vi "PicoScope4000aOpen.vi"(0 "error in (no error)":errorcluster, 1 "Serial Number":string, 2 "setProbeInteractionCallback":bool, 5 "Use Serial Number":bool, 7 "Resolution":u32(ring) items=["8-bit", "12-bit", "14-bit"], 9 "USB powered control":bool, 11 "USB 3.0 on non-USB 3.0 port control":bool) -> (4 "error out":errorcluster, 6 "handle":i16, 10 "Unit Info":T1, 12 "Max ADC value":i16, 13 "USB powered":bool, 14 "USB 3.0 on non-USB 3.0 port":bool)   [LabVIEW 2009]
doc: "This VI opens a PicoScope 3000a/b and returns a handle to the device."
uses:
  ps4000A.dll
  ps4000aWrap.dll
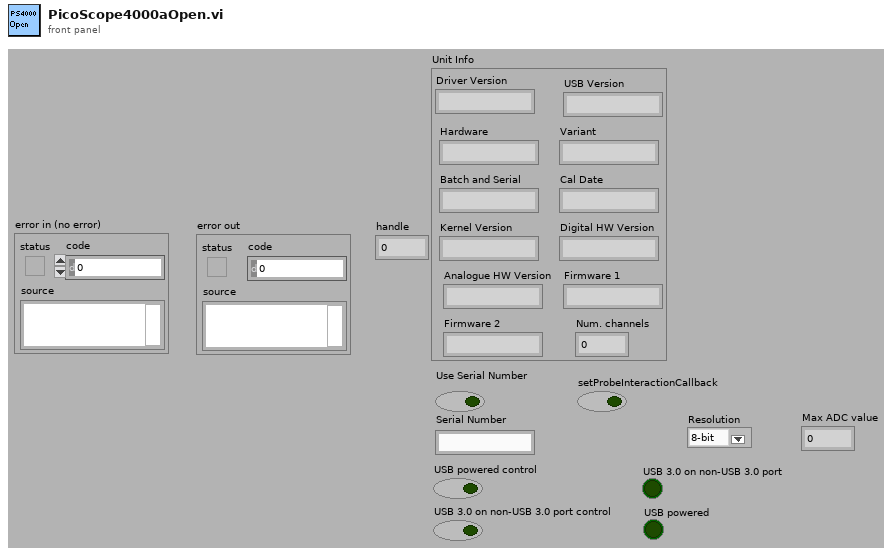
[diagram p1: front panel]
types:
  T1 = cluster{"Driver Version":string, "USB Version":string, "Hardware":string, "Variant":string, "Batch and Serial":string, "Cal Date":string, "Kernel Version":string, "Digital HW Version":string, "Analogue HW Version":string, "Firmware 1":string, "Firmware 2":string, "Num. channels":i16}
  T2 = cluster{"Driver Version":string, "USB Version":string, "Hardware":string, "Variant":string, "Batch and Serial":string, "Cal Date":string, "Kernel Version":string, "Digital HW Version":string, "Analogue HW Version":string, "Firmware 1":string, "Firmware 2":string}
  T3 = cluster{"Driver Version":string, "USB Version":string, "Hardware":string, "Variant":string, "Batch and Serial":string, "Cal Date":string, "Kernel Version":string, "Digital HW Version":string, "Analogue HW Version":string, "Firmware 1":string, "Firmware 2":string, i16}
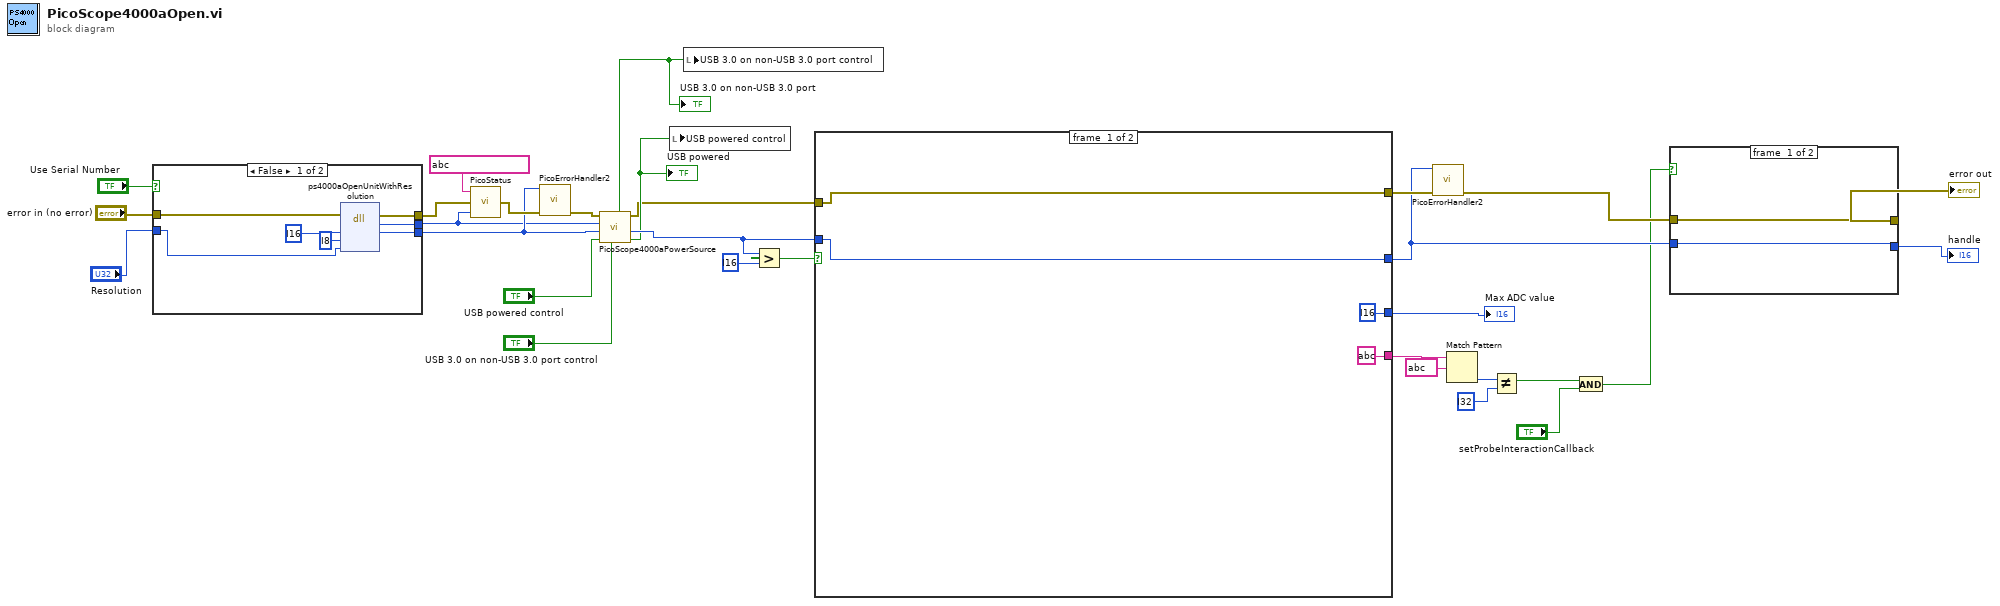
[diagram p0: block diagram]
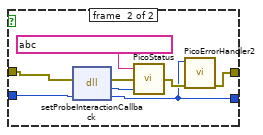
[diagram p2: hidden frame]
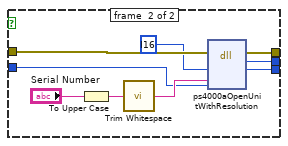
[diagram p3: hidden frame]
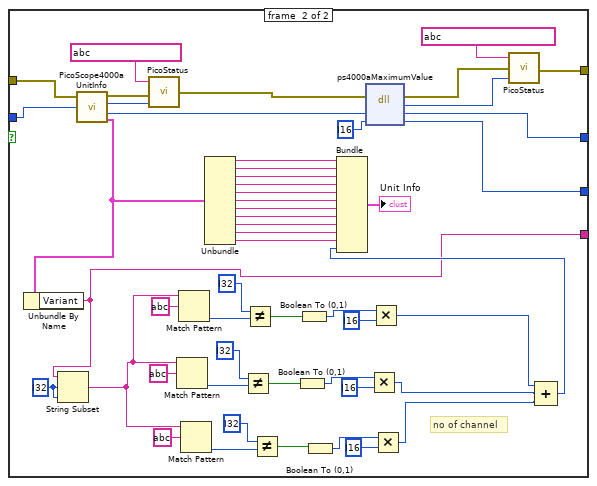
[diagram p4: hidden frame]
diagram:
  n1 = case shown="False" "Use Serial Number" {
    tunnel: "error in (no error)" -> [w37 w43]
    tunnel: [w36 w46] -> w17
    tunnel: [w35 w45] -> w15
    tunnel: [w34 w44] -> w16
    tunnel: "Resolution" -> [w31 w39]
    frame #0 {
      n2 = dll-call lib="ps4000A.dll" fn="ps4000aOpenUnitWithResolution" ("ps3000.dll:_ps3000_open_unit@0")(error in=w37, "handle"=i16 ?, "serial"=i8 ?, "resolution"=w31) -> (error out=w36:errorcluster, "PICO_STATUS"=w35:u32, "handle"=w34:i16)  [unwired: 4 in, 1 out]
    }
    frame #1 {
      n3 = To Upper Case(1:"Serial Number") -> (0:w41:string)
      n4 = call <vilib>:"Trim Whitespace.vi"("string"=w41) -> ("trimmed string"=w40:string)  [unwired: 1 in]
      n5 = dll-call lib="ps4000A.dll" fn="ps4000aOpenUnitWithResolution" ("ps3000.dll:_ps3000_open_unit@0")(error in=w43, "handle"=i16 ?, "serial"=w40, "resolution"=w39) -> (error out=w46:errorcluster, "PICO_STATUS"=w45:u32, "handle"=w44:i16)  [unwired: 4 in, 1 out]
    }
  }
  n6 = call "PicoStatus.vi"("PICO STATUS"=w15, "error in"=w17, "source"=string ?) -> ("error out"=w18:errorcluster)
  n7 = call "PicoErrorHandler2.vi"("error in (no error)"=w18, "handle In"=w16) -> ("error out"=w19:errorcluster)  [unwired: 9 in]
  n8 = call "PicoScope4000aPowerSource.vi"("USB 3.0 on non-USB 3.0 port control"="USB 3.0 on non-USB 3.0 port control", "USB powered control"="USB powered control", "handle in"=w16, "PICO STATUS IN"=w15, "error in (no error)"=w19) -> ("USB powered"=w21:bool, "handle out"=w26:i16, "error out"=w13:errorcluster, "USB 3.0 on non-USB 3.0 port"=w20:bool)  [unwired: 2 in, 1 out]
  "USB 3.0 on non-USB 3.0 port" <- w20
  "USB powered" <- w21
  n9 = local write "USB powered control"(w21) -> ()
  n10 = local write "USB 3.0 on non-USB 3.0 port control"(w20) -> ()
  n11 = Greater?(x=w26, y=i16 ?) -> (0:w29:bool)
  n12 = case shown="True" w29 {
    tunnel: w26 -> [w50 w101]
    tunnel: [w50 w57] -> w10
    tunnel: [w49 w61] -> w14
    tunnel: w13 -> [w49 w55]
    tunnel: [i16 ? ("value") w54] -> w12
    tunnel: [string ? ("Variant") w51] -> w7
    frame #0 {
    }
    frame #1 {
      w99 = i32 ? ("offset (0)")
      # "no of channel"
      n13 = call "PicoScope4000aUnitInfo.vi"("error in (no error)"=w55, "handle in"=w101) -> ("error out"=w100:errorcluster, "PICO_STATUS"=w52:u32, "handle out"=w56:i16, "Unit Info"=w98:T2)  [unwired: 1 in]
      n14 = Unbundle By Name(w98) -> ("Variant"=w51:string)
      n15 = String Subset(string=w51, offset (0)=w99, length (rest)=w99) -> (substring=w67:string)
      n16 = call "PicoStatus.vi"("PICO STATUS"=w52, "error in"=w100, "source"=string ?) -> ("error out"=w60:errorcluster)
      n17 = Match Pattern(string=w67, regular expression=string ?) -> (offset past match=w84:i32)  [unwired: 1 in, 3 out]
      n18 = Match Pattern(string=w67, regular expression=string ?) -> (offset past match=w72:i32)  [unwired: 1 in, 3 out]
      n19 = Match Pattern(string=w67, regular expression=string ?) -> (offset past match=w82:i32)  [unwired: 1 in, 3 out]
      n20 = Unbundle(w98) -> ("Driver Version"=w97:string, "USB Version"=w96:string, "Hardware"=w95:string, "Variant"=w94:string, "Batch and Serial"=w93:string, "Cal Date"=w92:string, "Kernel Version"=w91:string, "Digital HW Version"=w90:string, "Analogue HW Version"=w89:string, "Firmware 1"=w88:string, "Firmware 2"=w87:string)
      n21 = Not Equal?(x=i32 ?, y=w84) -> (x != y?=w80:bool)
      n22 = Not Equal?(x=i32 ?, y=w72) -> (x != y?=w70:bool)
      n23 = Not Equal?(x=i32 ?, y=w82) -> (x != y?=w79:bool)
      n24 = Boolean To (0,1)(Boolean=w80) -> (0, 1=w78:i16)
      n25 = Boolean To (0,1)(Boolean=w70) -> (0, 1=w69:i16)
      n26 = Boolean To (0,1)(Boolean=w79) -> (0, 1=w76:i16)
      n27 = dll-call lib="ps4000a.dll" fn="ps4000aMaximumValue"(error in=w60, "handle"=w56, "value"=i16 ?) -> (error out=w59:errorcluster, "PICO_STATUS"=w58:u32, "handle"=w57:i16, "value"=w54:i16)  [unwired: 2 in, 1 out]
      n28 = Multiply(x=w78, y=i16 ?) -> (x*y=w65:i16)
      n29 = Multiply(x=w69, y=i16 ?) -> (x*y=w66:i16)
      n30 = Multiply(x=w76, y=i16 ?) -> (x*y=w64:i16)
      n31 = call "PicoStatus.vi"("PICO STATUS"=w58, "error in"=w59, "source"=string ?) -> ("error out"=w61:errorcluster)
      n32 = Compound Arithmetic op=ADD(w66, w65, w64) -> (w63:i16)
      n33 = Bundle("Driver Version"=w97, "USB Version"=w96, "Hardware"=w95, "Variant"=w94, "Batch and Serial"=w93, "Cal Date"=w92, "Kernel Version"=w91, "Digital HW Version"=w90, "Analogue HW Version"=w89, "Firmware 1"=w88, "Firmware 2"=w87, w63) -> (→"Unit Info":T3)  [unwired: 1 in]
    }
  }
  "Max ADC value" <- w12
  n34 = call "PicoErrorHandler2.vi"("error in (no error)"=w14, "handle In"=w10) -> ("error out"=w11:errorcluster)  [unwired: 9 in]
  n35 = Match Pattern(string=w7, regular expression=string ?) -> (offset past match=w5:i32)  [unwired: 1 in, 3 out]
  n36 = Not Equal?(x=w5, y=i32 ?) -> (x != y?=w3:bool)
  n37 = And(x=w3, y="setProbeInteractionCallback") -> (x .and. y?=w1:bool)
  n38 = case shown="True" w1 {
    tunnel: w11 -> [w104 w112]
    tunnel: [w104 w106] -> w9
    tunnel: [w103 w105] -> w8
    tunnel: w10 -> [w103 w111]
    frame #0 {
    }
    frame #1 {
      n39 = dll-call lib="ps4000aWrap.dll" fn="setProbeInteractionCallback"(error in=w112, "handle"=w111) -> (error out=w110:errorcluster, "PICO_STATUS"=w108:u32, "handle"=w105:i16)  [unwired: 2 in, 1 out]
      n40 = call "PicoStatus.vi"("PICO STATUS"=w108, "error in"=w110, "source"=string ?) -> ("error out"=w107:errorcluster)
      n41 = call "PicoErrorHandler2.vi"("error in (no error)"=w107, "handle In"=w105) -> ("error out"=w106:errorcluster)  [unwired: 9 in]
    }
  }
  "handle" <- w8
  "error out" <- w9
